vi "Tosca-Synapse Thread.vi"(0 "IPC":T2, 7 "Data":T1) -> (8 "aborted":bool, 15 "error out":errorcluster)   [LabVIEW 2020]
uses:
  IPC VIs/Tosca-IPC.ctl
  Classes/Parameters/Parameters.lvclass
  Digital Input VIs/Tosca-DI Queue Data.ctl
  Digital Input VIs/Tosca-Input Event.ctl
  Digital Input VIs/Tosca-Input Criterion.ctl
  epl-vi-lib/Utility VIs/Type Defs/Logic State.ctl
  Typedefs/Tosca-Accumulator.ctl
  Typedefs/Tosca-State AODO.ctl
  Typedefs/Tosca-AO Runtime.ctl
  Typedefs/Tosca-DO Runtime.ctl
  epl-vi-lib/Signal Synthesis VIs/4th Generation/Classes/SignalManager/SignalManager.lvclass
  Typedefs/Tosca-Synapse Start Data.ctl
  IPC VIs/Tosca-Message.ctl
  IPC VIs/Tosca-Message Action.ctl
  Typedefs/Tosca-Thread Type.ctl
  Imaging VIs/Tosca-2P-Notifier Data.ctl
  Typedefs/Tosca-MATLAB Queue Data.ctl
  Visual Stim VIs/Tosca-Grating.ctl
  Visual Stim VIs/Tosca-Grating Type.ctl
  Typedefs/Tosca-File IO Notification.ctl
  epl-vi-lib/TCP VIs/TCP Params.ctl
  Tosca-Globals.vi
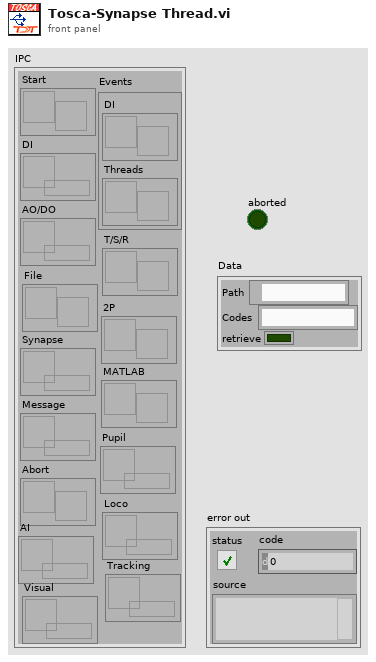
[diagram p1: front panel]
types:
  T1 = typedef "Tosca-Synapse Start Data.ctl" = cluster{"Path":path, "Codes":string, "retrieve":bool}
  T2 = typedef "Tosca-IPC.ctl" = cluster{"Start":refnum<notifier>, "DI":refnum<queue>, "AO/DO":refnum<queue>, "Synapse":refnum<queue>, "Message":refnum<queue>, "Abort":refnum<notifier>, "Events":cluster{"DI":refnum<user-event>, "Threads ":refnum<user-event>}, "T/S/R":refnum<notifier>, "2P":refnum<notifier>, "MATLAB":refnum<notifier>, "Pupil":refnum<queue>, "Loco":refnum<queue>, "AI":refnum<queue>, "Tracking":refnum<queue>, "Visual":refnum<queue>, "File":refnum<notifier>}
  T3 = enum16{"big-endian, network order", "native, host order", "little-endian"}
  T4 = typedef "TCP Params.ctl" = cluster{"IP Address":string, "Port":i32}
  T5 = typedef "Tosca-Thread Type.ctl" = enum16{"None", "AODO", "Masker", "ET", "Imaging", "Pupil", "AI", "DI", "Camera", "TTL out", "Loco", "Visual"}
  T6 = enum16{"open", "replace", "create", "open or create", "replace or create", "replace or create with confirmation"}
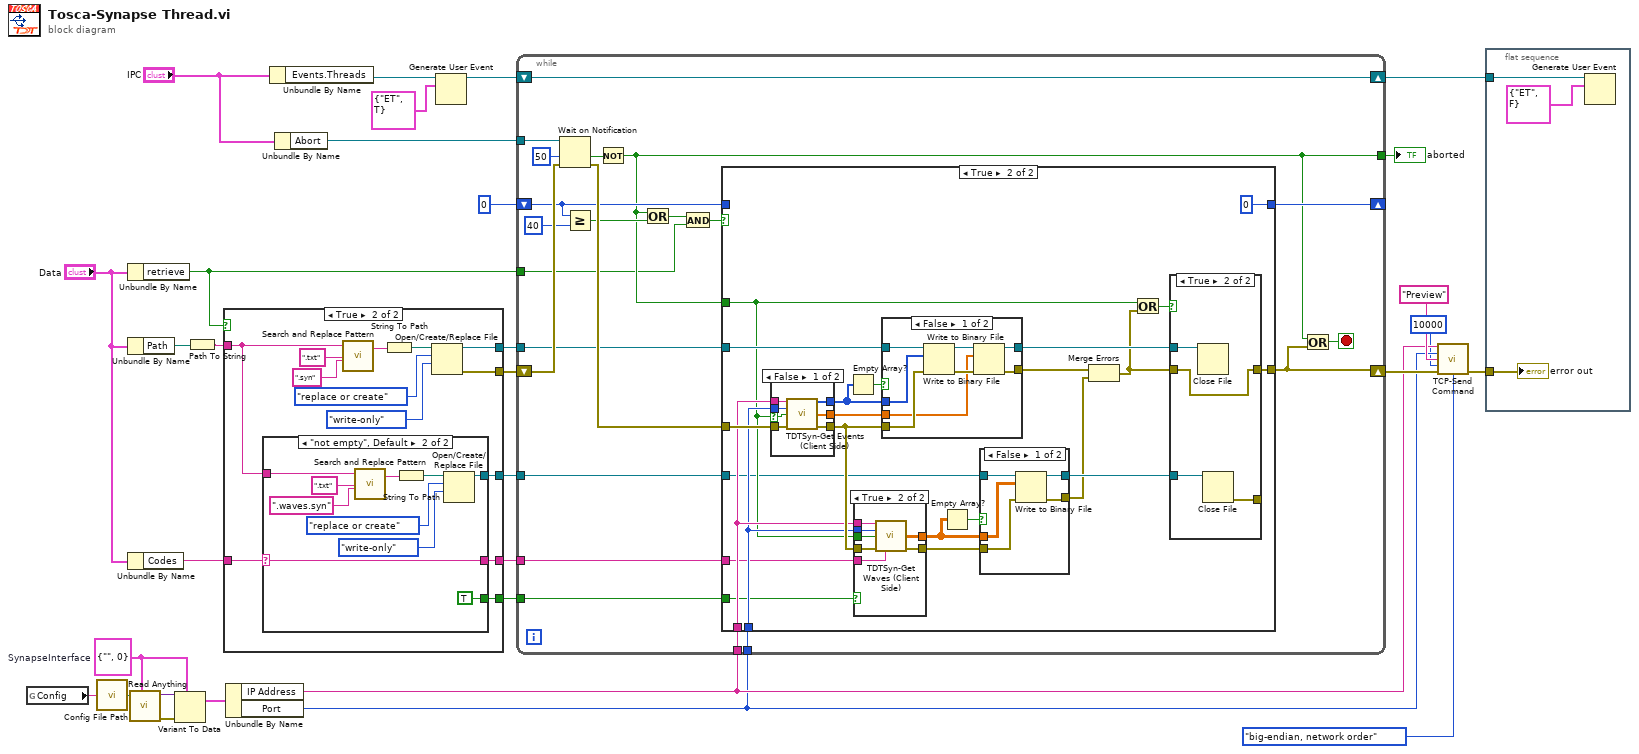
[diagram p0: block diagram]
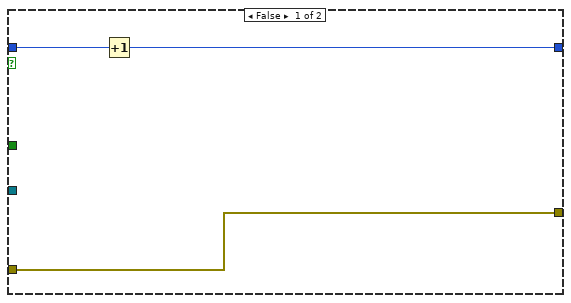
[diagram p4: hidden frame]
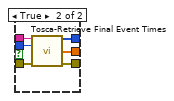
[diagram p7: hidden frame]
diagram:
  w24 = T4 {"IP Address"="", "Port"=0}  # SynapseInterface
  n1 = global read "Tosca-Globals.vi" "Config"() -> (w11:string)
  n2 = call "Config File Path.vi"("AppName"=w11) -> ("Default config file name"=w25:path)
  n3 = Unbundle By Name("Data") -> ("retrieve"=w10:bool)
  n4 = Unbundle By Name("Data") -> ("Path"=w9:path)
  n5 = Unbundle By Name("Data") -> ("Codes"=w6:string)
  n6 = call "Read Anything.vi"("Type of Anything"=w24, "Path (dialog)"=w25) -> ("Error Out"=w22:errorcluster, "Anything"=w23:variant)  [unwired: 7 in, 1 out]
  n7 = Variant To Data(error in=w22, type=w24, Variant=w23) -> (data=w21:T4)  [unwired: 1 out]
  n8 = Path To String(path=w9) -> (string=w8:string)
  n9 = case shown="True" w10 {
    tunnel: [_ w38] -> w19
    tunnel: [_ w37] -> w13
    tunnel: w8 -> [_ w35]
    tunnel: w6 -> [_ w36]
    tunnel: [_ w34] -> w5
    tunnel: [_ w33] -> w4
    tunnel: [_ w32] -> w3
    frame False {
    }
    frame True {
      n10 = case shown="\"not empty\", Default" w36 {
        selector: w36 -> [_ w46]
        tunnel: w35 -> [_ w48]
        tunnel: [_ w47] -> w34
        tunnel: [_ w46] -> w33
        tunnel: [_ TRUE] -> w32
        frame "" {
        }
        frame "not empty", Default {
          n11 = call <vilib>:"Search and Replace Pattern.vi"("string"=w48, "regular expression (\"\")"=".txt" ("regular expression (\"\")"), "replace string (\"\")"=".waves.syn" ("replace string (\"\")")) -> ("result string"=w52:string)  [unwired: 2 in, 1 out]
          n12 = String To Path(string=w52) -> (path=w51:path)
          n13 = Open/Create/Replace File(file path (use dialog)=w51, operation (0:open)=T6."replace or create", access (0:read/write)=enum16{"read/write", "read-only", "write-only"}."write-only") -> (refnum out=w47:refnum<file>)  [unwired: 3 in, 2 out]
        }
      }
      n14 = call <vilib>:"Search and Replace Pattern.vi"("string"=w35, "regular expression (\"\")"=".txt" ("regular expression (\"\")"), "replace string (\"\")"=".syn" ("replace string (\"\")")) -> ("result string"=w42:string)  [unwired: 2 in, 1 out]
      n15 = String To Path(string=w42) -> (path=w41:path)
      n16 = Open/Create/Replace File(file path (use dialog)=w41, operation (0:open)=T6."replace or create", access (0:read/write)=enum16{"read/write", "read-only", "write-only"}."write-only") -> (refnum out=w38:refnum<file>, error out=w37:errorcluster)  [unwired: 3 in, 1 out]
    }
  }
  n17 = Unbundle By Name(w21) -> ("IP Address"=w15:string, "Port"=w14:i32)
  n18 = Unbundle By Name("IPC") -> ("Events.Threads"=w31:refnum<user-event>)
  n19 = Unbundle By Name("IPC") -> ("Abort"=w27:refnum<notifier>)
  n20 = Generate User Event(user event=w31, event data cluster=cluster{"ID":T5, "Running":bool} {"ID"=enum."ET", "Running"=TRUE} ("event data")) -> (user event out=w29:refnum<user-event>)  [unwired: 2 in, 1 out]
  n21 = while {
    tunnel: w27 -> [w73]
    shift-right: [w76] -> w28
    shift-left: w29 -> [w76]
    shift-right: [w69] -> w18
    shift-left: w13 -> [w71]
    tunnel: w15 -> [w68]
    tunnel: w14 -> [w67]
    tunnel: w19 -> [w66]
    shift-right: [w64] -> _
    shift-left: 0 -> [w65]
    tunnel: [w60] -> w16
    tunnel: w10 -> [w58]
    tunnel: w5 -> [w56]
    tunnel: w4 -> [w57]
    tunnel: w3 -> [w55]
    stop <- w72 stop-if-true
    n22 = Wait on Notification(notifier=w73, timeout in ms (-1)=50, error in (no error)=w71) -> (timed out?=w75:bool, error out=w70:errorcluster)  [unwired: 1 in, 2 out]
    n23 = Greater Or Equal?(x=w65, y=40) -> (x >= y?=w63:bool)
    n24 = Not(x=w75) -> (.not. x?=w60:bool)
    n25 = Or(x=w60, y=w63) -> (x .or. y?=w62:bool)
    n26 = And(x=w62, y=w58) -> (x .and. y?=w61:bool)
    n27 = case shown="True" w61 {
      tunnel: w70 -> [w79 w100]
      tunnel: w60 -> [_ w90]
      tunnel: [w79 w102] -> w69
      tunnel: w68 -> [_ w92]
      tunnel: w67 -> [_ w91]
      tunnel: w66 -> [_ w95]
      tunnel: w65 -> [w78 _]
      tunnel: [w77 0] -> w64
      tunnel: w57 -> [_ w89]
      tunnel: w56 -> [_ w88]
      tunnel: w55 -> [_ w80]
      frame False {
        n28 = Increment(x=w78) -> (x+1=w77:i32)
      }
      frame True {
        n29 = case shown="False" w90 {
          selector: w90 -> [w123 _]
          tunnel: w92 -> [w122 w129]
          tunnel: w91 -> [w121 w128]
          tunnel: w100 -> [w120 w127]
          tunnel: [w119 w124] -> w93
          tunnel: [w118 w125] -> w99
          tunnel: [w117 w126] -> w97
          frame False {
            n30 = call "TDTSyn-Get Events (Client Side).vi"("IP Address"=w122, "Port"=w121, "last read"=w123, "error in (no error)"=w120) -> ("Codes"=w117:i16[], "Times"=w118:sgl[], "error out"=w119:errorcluster)  [unwired: 9 in]
          }
          frame True {
            n31 = call "Tosca-Retrieve Final Event Times.vi"("IP Address"=w129, "Port"=w128, "error in (no error)"=w127) -> ("Codes"=w126:i16[], "Times"=w125:sgl[], "error out"=w124:errorcluster)  [unwired: 10 in]
          }
        }
        n32 = Empty Array?(array=w97) -> (empty?=w98:bool)
        n33 = case shown="True" w80 {
          tunnel: w93 -> [_ w116]
          tunnel: w92 -> [_ w115]
          tunnel: w91 -> [_ w114]
          tunnel: w89 -> [_ w110]
          tunnel: [_ w113] -> w87
          tunnel: [_ w112] -> w86
          tunnel: w90 -> [_ w111]
          frame False {
          }
          frame True {
            n34 = call "TDTSyn-Get Waves (Client Side).vi"("IP Address"=w115, "Port"=w114, "last read"=w111, "error in (no error)"=w116, "Codes"=w110) -> ("waves"=w112:dbl[][], "error out"=w113:errorcluster)  [unwired: 9 in]
          }
        }
        n35 = case shown="False" w98 {
          tunnel: w93 -> [w136 w139]
          tunnel: w99 -> [w130 _]
          tunnel: w97 -> [w131 _]
          tunnel: [w132 w139] -> w96
          tunnel: w95 -> [w137 w138]
          tunnel: [w133 w138] -> w94
          frame False {
            n36 = Write to Binary File(file (use dialog)=w137, data=w131, error in=w136) -> (refnum out=w134:refnum<file>, error out=w135:errorcluster)  [unwired: 3 in, 1 out]
            n37 = Write to Binary File(file (use dialog)=w134, data=w130, error in=w135) -> (refnum out=w133:refnum<file>, error out=w132:errorcluster)  [unwired: 3 in, 1 out]
          }
          frame True {
          }
        }
        n38 = Empty Array?(array=w86) -> (empty?=w85:bool)
        n39 = case shown="False" w85 {
          tunnel: w87 -> [w106 w109]
          tunnel: w86 -> [w103 _]
          tunnel: [w104 w109] -> w83
          tunnel: w88 -> [w107 w108]
          tunnel: [w105 w108] -> w84
          frame False {
            n40 = Write to Binary File(file (use dialog)=w107, data=w103, error in=w106) -> (refnum out=w105:refnum<file>, error out=w104:errorcluster)  [unwired: 3 in, 1 out]
          }
          frame True {
          }
        }
        n41 = Merge Errors(w96, w83) -> (w81:errorcluster)
        n42 = Or(x=w90, y=w81) -> (x .or. y?=w82:bool)
        n43 = case shown="True" w82 {
          tunnel: w94 -> [_ w144]
          tunnel: [w140 w141] -> w102
          tunnel: w81 -> [w140 w141]
          tunnel: w84 -> [_ w143]
          tunnel: [_ w142] -> _
          frame False {
          }
          frame True {
            n44 = Close File(refnum=w144) -> ()  [unwired: 1 in, 2 out]
            n45 = Close File(refnum=w143) -> (error out=w142:errorcluster)  [unwired: 1 in, 1 out]
          }
        }
      }
    }
    n46 = Or(x=w60, y=w69) -> (x .or. y?=w72:bool)
  }
  "aborted" <- w16
  n47 = call "TCP-Send Command.vi"("PXI Address"=w15, "Port"=w14, "Command"="Preview", "timeout (ms)"=10000, "error in (no error)"=w18, "byte order"=T3."big-endian, network order") -> ("error out"=w2:errorcluster)  [unwired: 9 in]
  n48 = flat-sequence {
    tunnel: w28 -> [w147]
    tunnel: w2 -> [w145]
    frame #0 {
      n49 = Generate User Event(user event=w147, event data cluster=cluster{"ID":T5, "Running":bool} {"ID"=enum."ET", "Running"=FALSE} ("event data")) -> ()  [unwired: 2 in, 2 out]
      "error out" <- w145
    }
  }
